vi "CIPC_Double_Tag.vi"() -> (3 "CIF_CIPC_Chn_Double.lvclass":refnum<class "CIF_CIPC_Chn_Double.lvclass">)   [LabVIEW 2021, in "CIF_CIPC_Chn_Double.lvclass"]
uses:
  CIF_CIPC_Chn_Double.lvclass
  CIF_CIPC_Chn_Double.lvclass/CIF_CIPC_Chn_Double.ctl
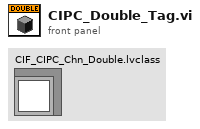
[diagram p1: front panel]
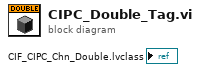
[diagram p0: block diagram]
diagram:
